vi "CST_ADSxxxx Register.vi"() -> (0 "ADC Register":T1 {"Base" format="%.0x"; "Item Count" format="%.0x"; "Value" format="%.0x"; "RegMap"."Mask" format="%.0x"; "Default" format="%.0x"; "Register" format="%.0x"})   [LabVIEW 2010]
uses:
  TYP_ADSxxxx Register.ctl
  TYP_RegMap Item.ctl
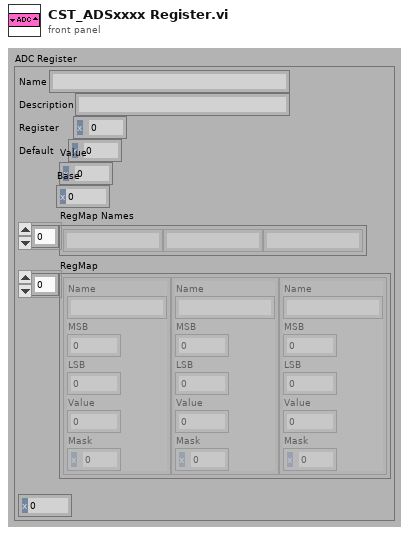
[diagram p1: front panel]
types:
  T1 = typedef "TYP_ADSxxxx Register.ctl" = cluster{"Name":string, "Description":string, "Register":u16, "Default":u16, "Value":u16, "Base":u16, "RegMap Names":string[], "RegMap":T2[], "Item Count":u8}
  T2 = typedef "TYP_RegMap Item.ctl" = cluster{"Name":string, "MSB":u16, "LSB":u16, "Value":u16, "Mask":u16}
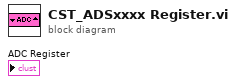
[diagram p0: block diagram]
diagram:
